vi "Templates Folder.vi"(3 "Relative Path (\"\")":string) -> (1 "Templates Folder":path)   [LabVIEW 2011]
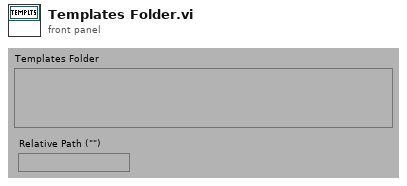
[diagram p1: front panel]
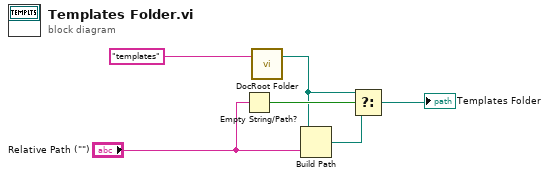
[diagram p0: block diagram]
diagram:
  n1 = Empty String/Path?(string/path="Relative Path (\"\")") -> (empty?=w5:bool)
  n2 = call "DocRoot Folder.vi"("Relative Path (\"\" - Folder)"="templates" ("name or relative path")) -> ("DocumentRoot Folder"=w1:path)  [unwired: 2 in]
  n3 = Build Path(base path=w1, name or relative path="Relative Path (\"\")") -> (appended path=w3:path)
  n4 = Select(t=w1, s=w5, f=w3) -> (s? t:f=→"Templates Folder":path)
